vi "findSharedBasePath.vi"(10 "arrayOfPaths":path[](array[path])) -> (2 "commonRootPath":path)   [LabVIEW 2021]
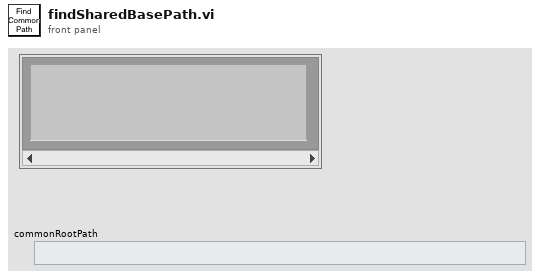
[diagram p1: front panel]
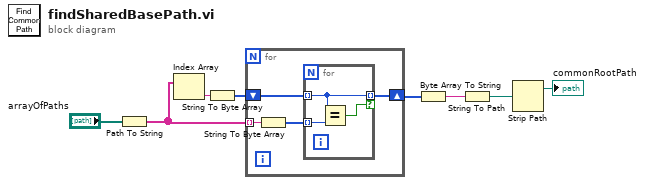
[diagram p0: block diagram]
diagram:
  n1 = Path To String(path="arrayOfPaths") -> (string=w7:string[])
  n2 = Index Array(array=w7) -> (element=w8:string)  [unwired: 1 in]
  n3 = String To Byte Array(string=w8) -> (unsigned byte array=w6:u8[])
  n4 = for {
    tunnel: w7 -> [w12] mode=indexing
    shift-right: [w9] -> w5
    shift-left: w6 -> [w10]
    n5 = String To Byte Array(string=w12) -> (unsigned byte array=w11:u8[])
    n6 = for {
      tunnel: w11 -> [w14] mode=indexing
      tunnel: w10 -> [w15] mode=indexing
      tunnel: [w15] -> w9 mode=indexing if=w13
      n7 = Equal?(x=w15, y=w14) -> (x = y?=w13:bool)
    }
  }
  n8 = Byte Array To String(unsigned byte array=w5) -> (string=w4:string)
  n9 = String To Path(string=w4) -> (path=w3:path)
  n10 = Strip Path(path=w3) -> (stripped path=→"commonRootPath":path)  [unwired: 1 out]
